vi "Add Missing Pin Error.vi"(8 "error in":errorcluster, 9 "instrument type id":string, 10 "site":i32, 11 "missing pin or relay names":string[](array[string])) -> (0 "error out":errorcluster)   [LabVIEW 2020, in "MeasurementLink Session Management.lvlib" / "Session Reservation.lvclass"]
uses:
  Session Reservation.lvclass
  MeasurementLink Measurement Server/Helpers/Error Strings Global Internal.vi
  Session Reservation.lvclass/Session Reservation.ctl
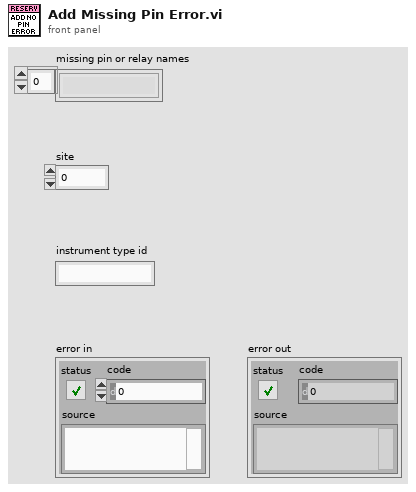
[diagram p1: front panel]
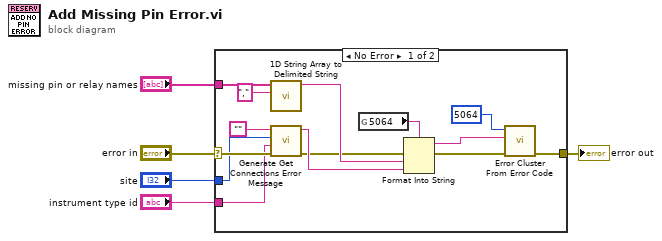
[diagram p0: block diagram]
diagram:
  n1 = case shown="No Error" "error in" {
    selector: "error in" -> [w11 w20]
    tunnel: [w19 w20] -> w4
    tunnel: "missing pin or relay names" -> [w14 _]
    tunnel: "site" -> [w10 _]
    tunnel: "instrument type id" -> [w9 _]
    frame No Error {
      n2 = call <vilib>:"1D String Array to Delimited String.vi"("delimiter"=",", "string array"=w14) -> ("delimited string"=w12:string)  [unwired: 9 in]
      n3 = call "Generate Get Connections Error Message.vi"("error in"=w11, "instrument type id"=w9, "site"=w10, "pin or relay names"="") -> ("error out"=w6:errorcluster, "error string"=w7:string)  [unwired: 6 in]
      n4 = global read "Error Strings Global Internal.vi" "5064"() -> (w18:string)
      n5 = Format Into String(format string=w18, error in=w6, w12, w7) -> (resulting string=w15:string, error out=w17:errorcluster)  [unwired: 1 in]
      n6 = call <vilib>:"Error Cluster From Error Code.vi"("error in (no error)"=w17, "error message (\"\")"=w15, "error code (0)"=5064) -> ("error out"=w19:errorcluster)  [unwired: 6 in]
    }
    frame Error {
    }
  }
  "error out" <- w4
